vi "Mitsubishi_Request Message Format.vi"(8 "error in":errorcluster, 11 "Request Message Format":T1={"Access Route"={"Network No."="\u0000", "PC No."="ÿ", "Module I/O No."="\u0003", "Module Station No."="\u0000"}, "Monitoring Timer(ms)"=4000, "Request Type"=enum."Batch read in word units", "Request Data"=variant}) -> (0 "error out":errorcluster, 2 "Byte To Read":i32, 3 "Request Message":string)   [LabVIEW 2018]
uses:
  Data Def/Mitsubishi_Request Message Format.ctl
  Data Def/Mitsubishi_Access Route.ctl
  Data Def/Mitsubishi_Request Type.ctl
  Data Def/Mitsubishi_Batch Read In Word Units Command.ctl
  Data Def/Mitsubishi_Device Code.ctl
  Data Def/Mitsubishi_Registers Data Type.ctl
  Data Def/Mitsubishi_Batch Write In Word Units Command.ctl
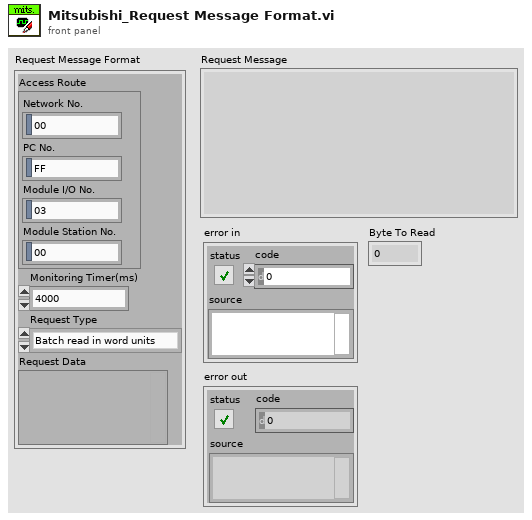
[diagram p1: front panel]
types:
  T1 = typedef "Mitsubishi_Request Message Format.ctl" = cluster{"Access Route":T2, "Monitoring Timer(ms)":u16, "Request Type":T3, "Request Data":variant}
  T2 = typedef "Mitsubishi_Access Route.ctl" = cluster{"Network No.":string, "PC No.":string, "Module I/O No.":string, "Module Station No.":string}
  T3 = typedef "Mitsubishi_Request Type.ctl" = enum16{"Batch read in word units", "Batch write in word units"}
  T4 = typedef "Mitsubishi_Batch Read In Word Units Command.ctl" = cluster{"Head Device Number":u16, "Device Code":T5, "Number Of Device Point":u16, "Registers Data Type":T6}
  T5 = typedef "Mitsubishi_Device Code.ctl" = u8
  T6 = typedef "Mitsubishi_Registers Data Type.ctl" = enum16{"16 Bit int", "16 Bit Uint", "32 Bit int", "32 Bit Uint", "32 Bit float", "64 Bit double", "Characters"}
  T7 = typedef "Mitsubishi_Batch Write In Word Units Command.ctl" = cluster{"Head Device Number":u16, "Device Code":T5, "Write Data":i16[]}
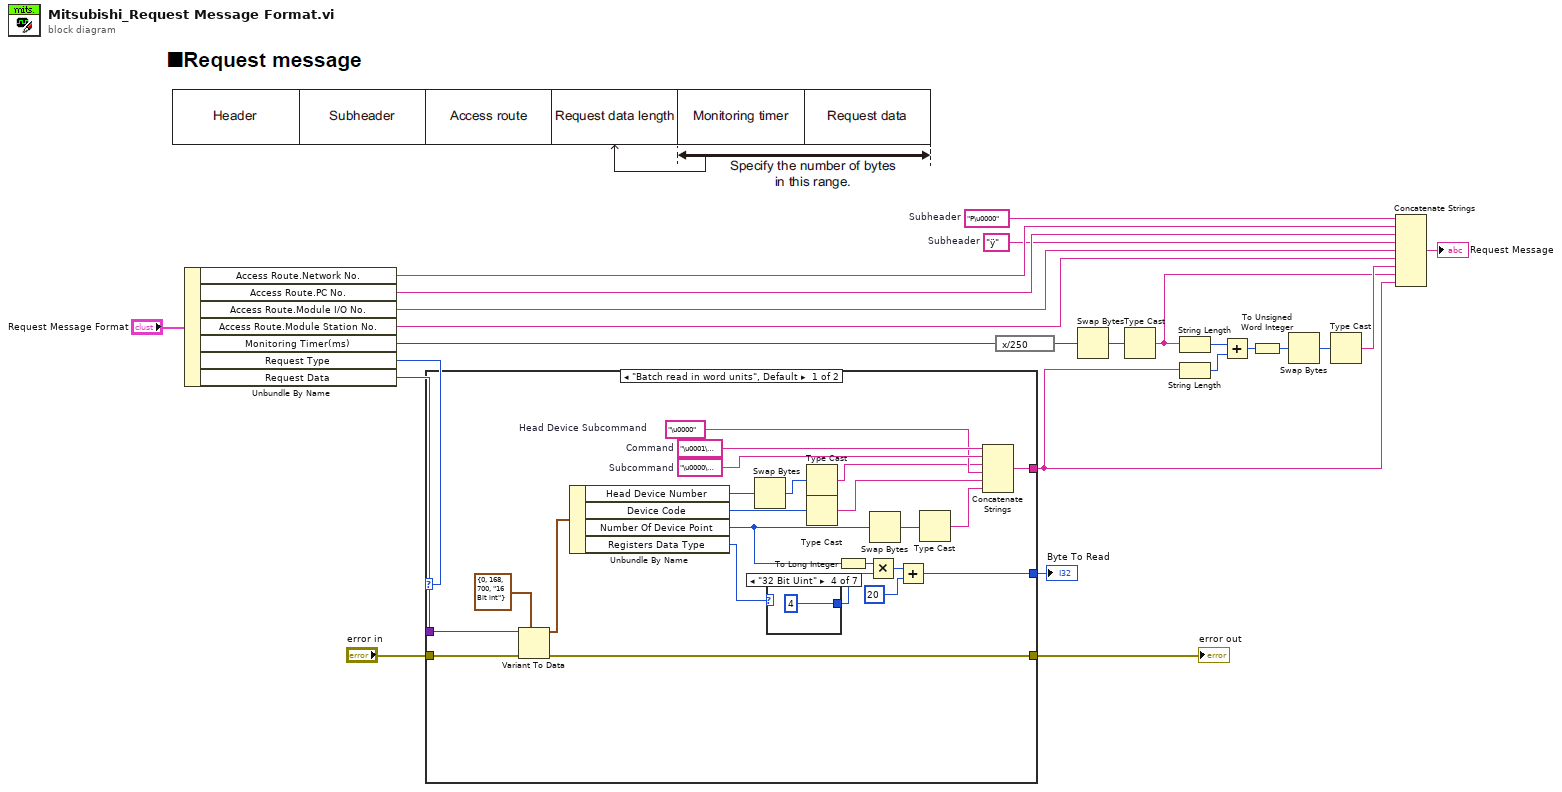
[diagram p0: block diagram]
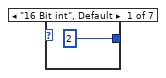
[diagram p2: hidden frame]
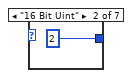
[diagram p3: hidden frame]
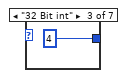
[diagram p4: hidden frame]
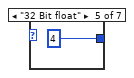
[diagram p5: hidden frame]
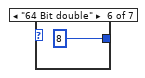
[diagram p6: hidden frame]
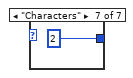
[diagram p7: hidden frame]
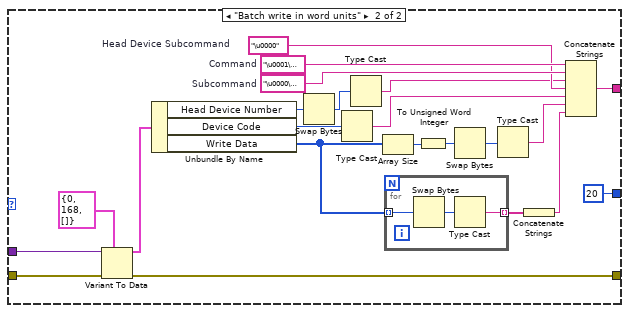
[diagram p8: hidden frame]
diagram:
  w9 = "ÿ"  # Subheader
  w16 = "P\u0000"  # Subheader
  n1 = Unbundle By Name("Request Message Format") -> ("Access Route.Network No."=w15:string, "Access Route.PC No."=w14:string, "Access Route.Module I/O No."=w8:string, "Access Route.Module Station No."=w7:string, "Monitoring Timer(ms)"=w18:u16, "Request Type"=w23:T3, "Request Data"=w22:variant)
  n2 = case shown="\"Batch read in word units\", Default" w23 {
    tunnel: w22 -> [w47 w76]
    tunnel: "error in" -> [w46 w75]
    tunnel: [w34 w70] -> w4
    tunnel: [w33 20] -> w1
    tunnel: [w32 w69] -> w17
    frame "Batch read in word units", Default {
      w31 = "\u0000"  # Head Device Subcommand
      w44 = "\u0001\u0004"  # Command
      w43 = "\u0000\u0000"  # Subcommand
      n3 = Variant To Data(error in=w46, type=T4 {"Head Device Number"=0, "Device Code"=168, "Number Of Device Point"=700, "Registers Data Type"=enum."16 Bit int"} ("Batch Read In Word Units"), Variant=w47) -> (data=w28:T4, error out=w32:errorcluster)
      n4 = Unbundle By Name(w28) -> ("Head Device Number"=w27:u16, "Device Code"=w42:T5, "Number Of Device Point"=w35:u16, "Registers Data Type"=w36:T6)
      n5 = Swap Bytes(anything=w27) -> (byte swapped=w26:u16)
      n6 = case shown="\"32 Bit Uint\"" w36 {
        tunnel: [2 ("y") 2 ("y") 4 ("y") 4 ("y") 4 ("y") 8 ("y") 2 ("y")] -> w39
        frame "16 Bit int", Default {
        }
        frame "16 Bit Uint" {
        }
        frame "32 Bit int" {
        }
        frame "32 Bit Uint" {
        }
        frame "32 Bit float" {
        }
        frame "64 Bit double" {
        }
        frame "Characters" {
        }
      }
      n7 = Type Cast(x=w26) -> (*(type *) &x=w25:string)  [unwired: 1 in]
      n8 = Type Cast(x=w42) -> (*(type *) &x=w30:string)  [unwired: 1 in]
      n9 = To Long Integer(number=w35) -> (32bit integer=w40:i32)
      n10 = Multiply(x=w40, y=w39) -> (x*y=w37:i32)
      n11 = Swap Bytes(anything=w35) -> (byte swapped=w41:u16)
      n12 = Add(x=w37, y=20) -> (x+y=w33:i32)
      n13 = Type Cast(x=w41) -> (*(type *) &x=w29:string)  [unwired: 1 in]
      n14 = Concatenate Strings(w44, w43, w25, w31, w30, w29) -> (w34:string)
    }
    frame "Batch write in word units" {
      w68 = "\u0000"  # Head Device Subcommand
      w74 = "\u0001\u0014"  # Command
      w73 = "\u0000\u0000"  # Subcommand
      n15 = Variant To Data(error in=w75, type=T7 {"Head Device Number"=0, "Device Code"=168, "Write Data"=[]} ("Batch Write In Word Units"), Variant=w76) -> (data=w66:T7, error out=w69:errorcluster)
      n16 = Unbundle By Name(w66) -> ("Head Device Number"=w57:u16, "Device Code"=w72:T5, "Write Data"=w64:i16[])
      n17 = Swap Bytes(anything=w57) -> (byte swapped=w56:u16)
      n18 = Type Cast(x=w72) -> (*(type *) &x=w60:string)  [unwired: 1 in]
      n19 = Type Cast(x=w56) -> (*(type *) &x=w55:string)  [unwired: 1 in]
      n20 = Array Size(array=w64) -> (size(s)=w59:i32)
      n21 = for {
        tunnel: w64 -> [w78] mode=indexing
        tunnel: [w79] -> w63 mode=indexing
        n22 = Swap Bytes(anything=w78) -> (byte swapped=w77:i16)
        n23 = Type Cast(x=w77) -> (*(type *) &x=w79:string)  [unwired: 1 in]
      }
      n24 = To Unsigned Word Integer(number=w59) -> (unsigned 16bit integer=w58:u16)
      n25 = Swap Bytes(anything=w58) -> (byte swapped=w71:u16)
      n26 = Type Cast(x=w71) -> (*(type *) &x=w67:string)  [unwired: 1 in]
      n27 = Concatenate Strings(w63) -> (w62:string)
      n28 = Concatenate Strings(w74, w73, w55, w68, w60, w67, w62) -> (w70:string)
    }
  }
  "error out" <- w17
  "Byte To Read" <- w1
  n29 = expression code="x/250"(w18) -> (w19:u16)
  n30 = Swap Bytes(anything=w19) -> (byte swapped=w20:u16)
  n31 = Type Cast(x=w20) -> (*(type *) &x=w5:string)  [unwired: 1 in]
  n32 = String Length(string=w5) -> (length=w13:i32)
  n33 = String Length(string=w4) -> (length=w12:i32)
  n34 = Add(x=w13, y=w12) -> (x+y=w11:i32)
  n35 = To Unsigned Word Integer(number=w11) -> (unsigned 16bit integer=w3:u16)
  n36 = Swap Bytes(anything=w3) -> (byte swapped=w2:u16)
  n37 = Type Cast(x=w2) -> (*(type *) &x=w6:string)  [unwired: 1 in]
  n38 = Concatenate Strings(w16, w15, w14, w9, w8, w7, w6, w5, w4) -> (→"Request Message":string)
